vi "Select the Process Variable.vi"(9 "type":string, 10 "force":dbl, 11 "diameter":dbl) -> (3 "process variable":dbl)   [LabVIEW 2020]
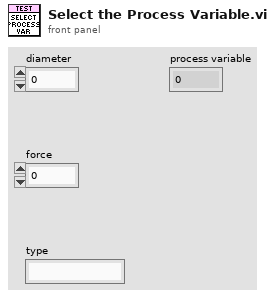
[diagram p1: front panel]
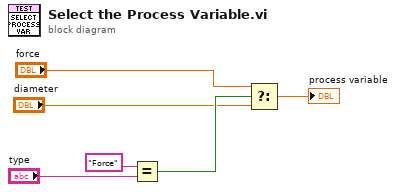
[diagram p0: block diagram]
diagram:
  n1 = Equal?(x="Force", y="type") -> (x = y?=w4:bool)
  n2 = Select(t="force", s=w4, f="diameter") -> (s? t:f=→"process variable":dbl)
